vi "reset AO.vi"() -> ()   [LabVIEW 2012]
doc: "SciScan 1.0 151216"
uses:
  <vilib>/DAQmx/write.llb/DAQmx Write (Analog DBL 1Chan 1Samp).vi
  <vilib>/DAQmx/write.llb/DAQmx Write (Analog 1D DBL NChan 1Samp).vi
  GFG/GFGbooleanGet.vi
  GFG/GFGnumericGet.vi
  GFG/GFGstringGet.vi
  <vilib>/DAQmx/create/channels.llb/DAQmx Create Channel (AO-Voltage-Basic).vi
  <vilib>/DAQmx/miscellaneous.llb/DAQmx Fill In Error Info.vi
  <vilib>/Utility/config.llb/Read Key (Double).vi
  <vilib>/Utility/config.llb/Read Key (String).vi
  GFG/GFG library.lvlib
  <vilib>/Utility/config.llb/NI_LVConfig.lvlib
panel:
  out "error out 3":errorcluster
  out "error out 2":errorcluster
  out "error out":errorcluster
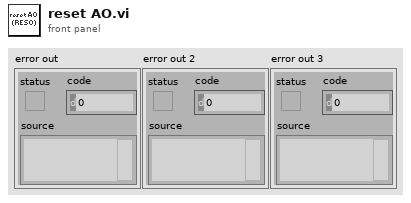
[diagram p1: front panel]
types:
  T1 = typedef "NI_LVConfig.lvlib/Config Data RefNum.ctl" = refnum<k1>
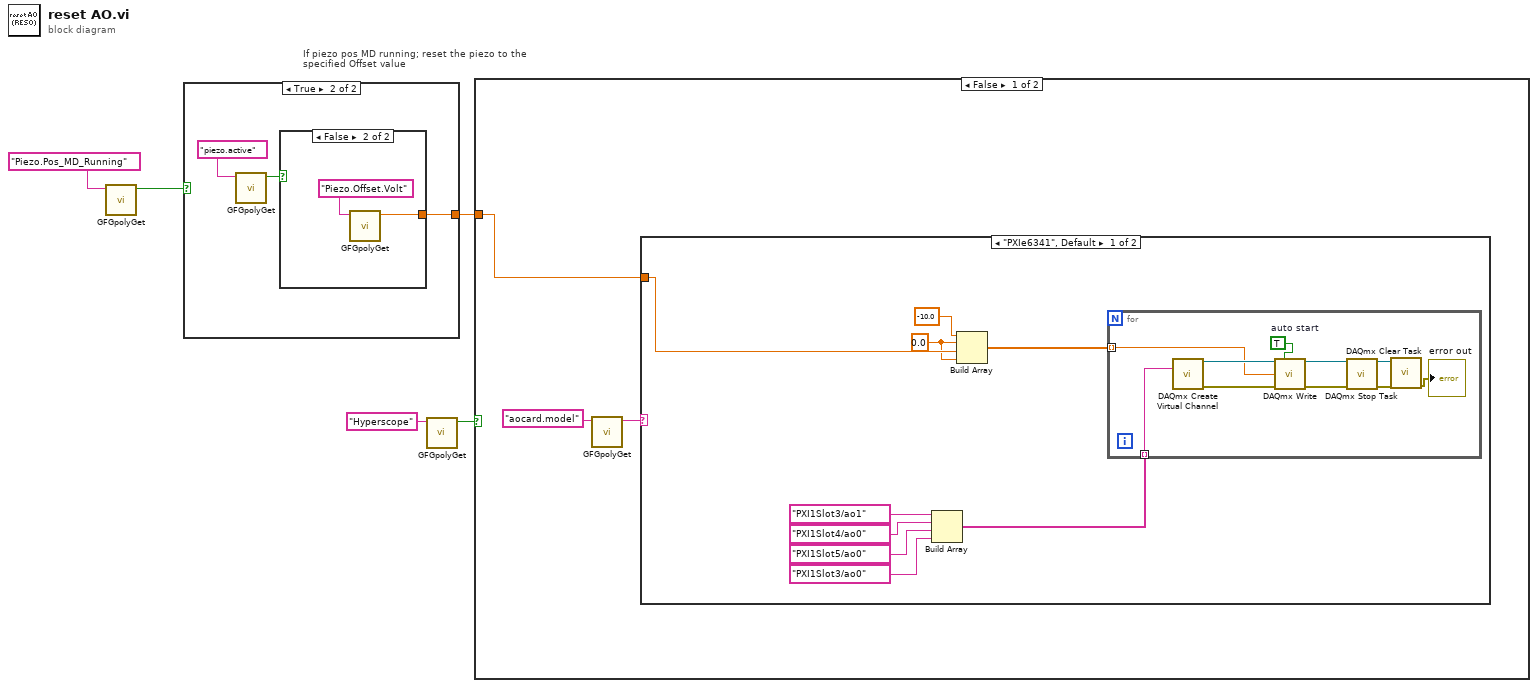
[diagram p0: block diagram]
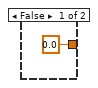
[diagram p2: hidden frame]
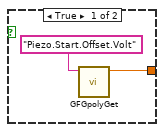
[diagram p3: hidden frame]
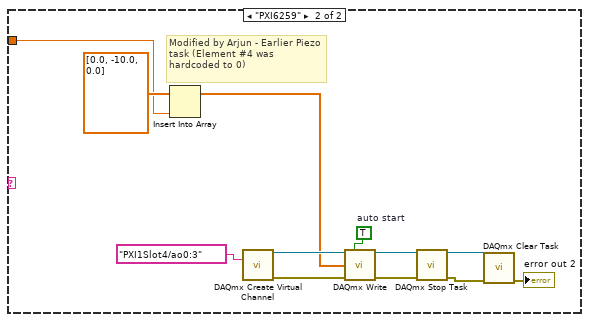
[diagram p4: hidden frame]
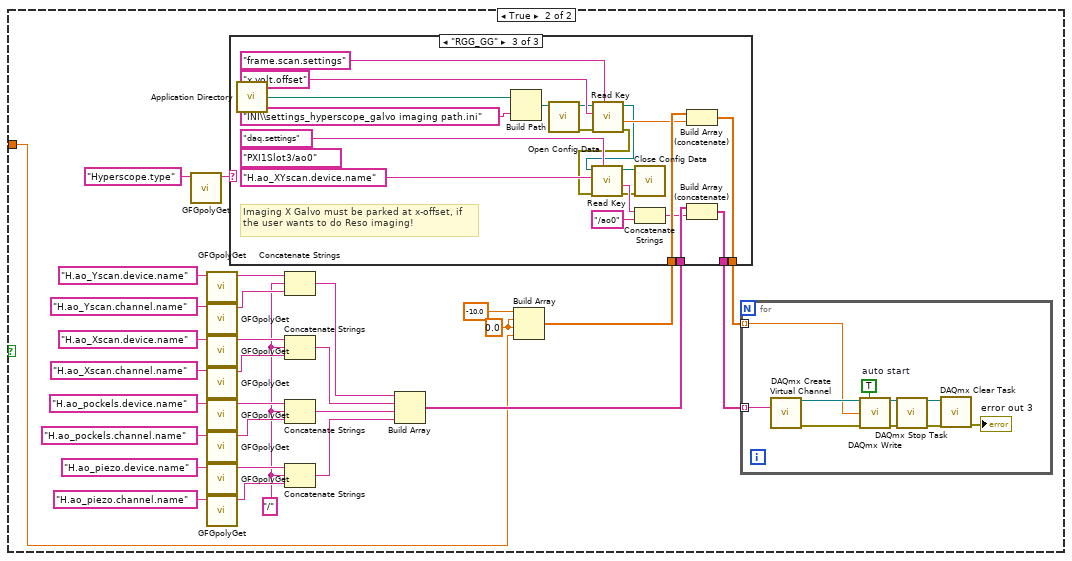
[diagram p5: hidden frame]
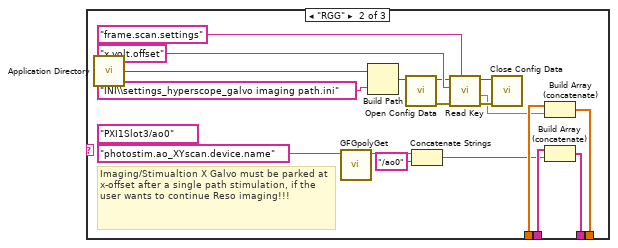
[diagram p7: hidden frame]
diagram:
  n1 = call-poly "GFGpolyGet.vi"("Variable Name in"="Piezo.Pos_MD_Running") -> ("Boolean Value OUT"=w2:bool)  [unwired: 9 in, 1 out]
  n2 = case "If piezo pos MD running; reset the piezo to the specified Offset value" shown="True" w2 {
    tunnel: [0.0 ("Numeric") w9] -> w1
    frame False {
    }
    frame True {
      n3 = call-poly "GFGpolyGet.vi"("Variable Name in"="piezo.active") -> ("Boolean Value OUT"=w7:bool)  [unwired: 9 in, 1 out]
      n4 = case shown="False" w7 {
        tunnel: [w10 w12] -> w9
        frame True {
          n5 = call-poly "GFGpolyGet.vi"("Variable Name in"="Piezo.Start.Offset.Volt") -> ("Numeric"=w10:dbl)  [unwired: 8 in, 2 out]
        }
        frame False {
          n6 = call-poly "GFGpolyGet.vi"("Variable Name in"="Piezo.Offset.Volt") -> ("Numeric"=w12:dbl)  [unwired: 8 in, 2 out]
        }
      }
    }
  }
  n7 = call-poly "GFGpolyGet.vi"("Variable Name in"="Hyperscope") -> ("Boolean Value OUT"=w4:bool)  [unwired: 9 in, 1 out]
  n8 = case shown="False" w4 {
    tunnel: w1 -> [w14 w48]
    frame False {
      n9 = call-poly "GFGpolyGet.vi"("Variable Name in"="aocard.model") -> ("String"=w15:string)  [unwired: 9 in, 1 out]
      n10 = case shown="\"PXIe6341\", Default" w15 {
        tunnel: w14 -> [w18 w36]
        frame "PXIe6341", Default {
          w17 = 0.0 ("element")
          n11 = Build Array(tag "PXI1Slot3/ao1" ("physical channels"), tag "PXI1Slot4/ao0" ("physical channels"), tag "PXI1Slot5/ao0" ("physical channels"), tag "PXI1Slot3/ao0" ("element")) -> (w19:tag[])
          n12 = Build Array(-10.0 ("data"), w17, w18, w17) -> (w20:dbl[])
          n13 = for {
            tunnel: w19 -> [w30] mode=indexing
            tunnel: w20 -> [w29] mode=indexing
            w33 = TRUE  # auto start
            n14 = call-poly <vilib>:"DAQmx Create Virtual Channel.vi"("physical channels"=w30) -> ("task out"=w34:refnum<k21>, "error out"=w32:errorcluster)  [unwired: 13 in]
            n15 = call-poly <vilib>:"DAQmx Write.vi"("task/channels in"=w34, "auto start"=w33, "data"=w29, "error in"=w32) -> ("task out"=w35:refnum<k21>, "error out"=w31:errorcluster)  [unwired: 9 in, 1 out]
            n16 = call <vilib>:"DAQmx Stop Task.vi"("task/channels in"=w35, "error in"=w31) -> ("task out"=w27:refnum<k21>, "error out"=w28:errorcluster)  [unwired: 12 in]
            n17 = call <vilib>:"DAQmx Clear Task.vi"("task in"=w27, "error in"=w28) -> ("error out"=→"error out":errorcluster)  [unwired: 13 in]
          }
        }
        frame "PXI6259" {
          w45 = TRUE  # auto start
          # "Modified by Arjun - Earlier Piezo task (Element #4 was hardcoded to 0)"
          n18 = Insert Into Array(array=dbl[] [0.0, -10.0, 0.0] ("data"), new element=w36) -> (w37:dbl[])  [unwired: 1 in]
          n19 = call-poly <vilib>:"DAQmx Create Virtual Channel.vi"("physical channels"=tag "PXI1Slot4/ao0:3") -> ("task out"=w46:refnum<k21>, "error out"=w44:errorcluster)  [unwired: 13 in]
          n20 = call-poly <vilib>:"DAQmx Write.vi"("task/channels in"=w46, "auto start"=w45, "data"=w37, "error in"=w44) -> ("task out"=w47:refnum<k21>, "error out"=w43:errorcluster)  [unwired: 9 in, 1 out]
          n21 = call <vilib>:"DAQmx Stop Task.vi"("task/channels in"=w47, "error in"=w43) -> ("task out"=w40:refnum<k21>, "error out"=w41:errorcluster)  [unwired: 12 in]
          n22 = call <vilib>:"DAQmx Clear Task.vi"("task in"=w40, "error in"=w41) -> ("error out"=→"error out 2":errorcluster)  [unwired: 13 in]
        }
      }
    }
    frame True {
      w55 = 0.0 ("element")
      w61 = "/" ("string")
      n23 = call-poly "GFGpolyGet.vi"("Variable Name in"="Hyperscope.type") -> ("String"=w53:string)  [unwired: 9 in, 1 out]
      n24 = call-poly "GFGpolyGet.vi"("Variable Name in"="H.ao_Yscan.device.name") -> ("String"=w73:string)  [unwired: 9 in, 1 out]
      n25 = call-poly "GFGpolyGet.vi"("Variable Name in"="H.ao_Yscan.channel.name") -> ("String"=w70:string)  [unwired: 9 in, 1 out]
      n26 = call-poly "GFGpolyGet.vi"("Variable Name in"="H.ao_Xscan.device.name") -> ("String"=w74:string)  [unwired: 9 in, 1 out]
      n27 = call-poly "GFGpolyGet.vi"("Variable Name in"="H.ao_Xscan.channel.name") -> ("String"=w77:string)  [unwired: 9 in, 1 out]
      n28 = call-poly "GFGpolyGet.vi"("Variable Name in"="H.ao_pockels.device.name") -> ("String"=w69:string)  [unwired: 9 in, 1 out]
      n29 = call-poly "GFGpolyGet.vi"("Variable Name in"="H.ao_pockels.channel.name") -> ("String"=w68:string)  [unwired: 9 in, 1 out]
      n30 = call-poly "GFGpolyGet.vi"("Variable Name in"="H.ao_piezo.device.name") -> ("String"=w66:string)  [unwired: 9 in, 1 out]
      n31 = call-poly "GFGpolyGet.vi"("Variable Name in"="H.ao_piezo.channel.name") -> ("String"=w67:string)  [unwired: 9 in, 1 out]
      n32 = Concatenate Strings(w73, w61, w70) -> (w60:string)
      n33 = Concatenate Strings(w74, w61, w77) -> (w59:string)
      n34 = Concatenate Strings(w69, w61, w68) -> (w58:string)
      n35 = Concatenate Strings(w66, w61, w67) -> (w57:string)
      n36 = Build Array(w60, w59, w58, w57) -> (w51:string[])
      n37 = Build Array(-10.0 ("data"), w55, w55, w48) -> (w52:dbl[])
      n38 = case shown="\"RGG_GG\"" w53 {
        tunnel: w52 -> [w79 w85 w110]
        tunnel: w51 -> [w78 w83 w104]
        tunnel: [w78 w81 w102] -> w49
        tunnel: [w79 w80 w108] -> w50
        frame Default {
          # "No additonal action required for these DAQ options."
        }
        frame "RGG" {
          (unwired) tag "PXI1Slot3/ao0"
          # "Imaging/Stimualtion X Galvo must be parked at x-offset after a single path stimulation, if the user wants to continue Reso imaging!!!"
          n39 = call <vilib>:"Application Directory.vi"() -> ("Application Directory"=w86:path)
          n40 = call-poly "GFGpolyGet.vi"("Variable Name in"="photostim.ao_XYscan.device.name") -> ("String"=w96:string)  [unwired: 9 in, 1 out]
          n41 = Build Path(base path=w86, name or relative path="INI\\settings_hyperscope_galvo imaging path.ini") -> (appended path=w87:path)
          n42 = call <vilib>:"Open Config Data.vi"("configuration file path"=w87) -> ("error out"=w89:errorcluster, "refnum"=w88:T1)  [unwired: 8 in, 1 out]
          n43 = Concatenate Strings(w96, "/ao0" ("string")) -> (w82:string)
          n44 = call-poly <vilib>:"Read Key.vi"("section"="frame.scan.settings" ("name or relative path"), "error in (no error)"=w89, "key"="x.volt.offset" ("name or relative path"), "refnum"=w88) -> ("error out"=w91:errorcluster, "value"=w84:dbl, "refnum out"=w90:T1)  [unwired: 4 in, 1 out]
          n45 = call <vilib>:"Close Config Data.vi"("error in (no error)"=w91, "refnum"=w90) -> ()  [unwired: 8 in, 2 out]
          n46 = Build Array (concatenate)(w85, w84) -> (w80:dbl[])
          n47 = Build Array (concatenate)(w83, w82) -> (w81:string[])
        }
        frame "RGG_GG" {
          (unwired) tag "PXI1Slot3/ao0"
          # "Imaging X Galvo must be parked at x-offset, if the user wants to do Reso imaging!"
          n48 = call <vilib>:"Application Directory.vi"() -> ("Application Directory"=w111:path)
          n49 = Build Path(base path=w111, name or relative path="INI\\settings_hyperscope_galvo imaging path.ini") -> (appended path=w112:path)
          n50 = call <vilib>:"Open Config Data.vi"("configuration file path"=w112) -> ("error out"=w114:errorcluster, "refnum"=w113:T1)  [unwired: 8 in, 1 out]
          n51 = call-poly <vilib>:"Read Key.vi"("section"="frame.scan.settings" ("name or relative path"), "error in (no error)"=w114, "key"="x.volt.offset" ("name or relative path"), "refnum"=w113) -> ("error out"=w100:errorcluster, "value"=w109:dbl, "refnum out"=w101:T1)  [unwired: 4 in, 1 out]
          n52 = call-poly <vilib>:"Read Key.vi"("section"="daq.settings" ("name or relative path"), "error in (no error)"=w100, "key"="H.ao_XYscan.device.name" ("Variable Name in"), "refnum"=w101) -> ("error out"=w98:errorcluster, "value"=w105:string, "refnum out"=w99:T1)  [unwired: 4 in, 1 out]
          n53 = call <vilib>:"Close Config Data.vi"("error in (no error)"=w98, "refnum"=w99) -> ()  [unwired: 8 in, 2 out]
          n54 = Concatenate Strings(w105, "/ao0" ("string")) -> (w103:string)
          n55 = Build Array (concatenate)(w110, w109) -> (w108:dbl[])
          n56 = Build Array (concatenate)(w104, w103) -> (w102:string[])
        }
      }
      n57 = for {
        tunnel: w50 -> [w123] mode=indexing
        tunnel: w49 -> [w120] mode=indexing
        w126 = TRUE  # auto start
        n58 = call-poly <vilib>:"DAQmx Create Virtual Channel.vi"("physical channels"=w120) -> ("task out"=w127:refnum<k21>, "error out"=w125:errorcluster)  [unwired: 13 in]
        n59 = call-poly <vilib>:"DAQmx Write.vi"("task/channels in"=w127, "auto start"=w126, "data"=w123, "error in"=w125) -> ("task out"=w128:refnum<k21>, "error out"=w124:errorcluster)  [unwired: 9 in, 1 out]
        n60 = call <vilib>:"DAQmx Stop Task.vi"("task/channels in"=w128, "error in"=w124) -> ("task out"=w121:refnum<k21>, "error out"=w122:errorcluster)  [unwired: 12 in]
        n61 = call <vilib>:"DAQmx Clear Task.vi"("task in"=w121, "error in"=w122) -> ("error out"=→"error out 3":errorcluster)  [unwired: 13 in]
      }
    }
  }
